vi "Create.vi"(5 "Test Executor in":refnum<class "Test Executor.lvclass">, 8 "error in (no error)":errorcluster, 11 "Application":refnum<vi>) -> (0 "error out":errorcluster, 3 "Test Executor":refnum<class "Test Executor.lvclass">)   [LabVIEW 2017, in "Test Executor.lvclass"]
uses:
  Test Executor.lvclass
  Test Executor.lvclass/Test Executor.ctl
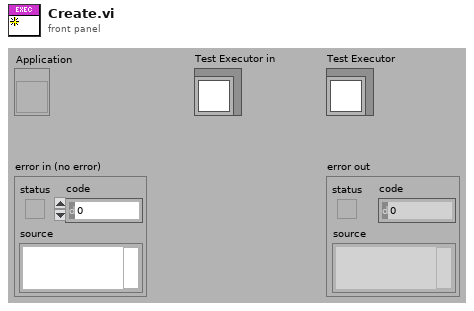
[diagram p1: front panel]
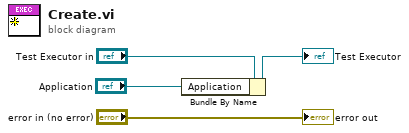
[diagram p0: block diagram]
diagram:
  n1 = Bundle By Name(cluster="Test Executor in", "Application"="Application") -> (→"Test Executor":refnum<class "Test Executor.lvclass">)
  "error out" <- "error in (no error)"
